vi "GetDecorationName.vi"(6 "error in":errorcluster, 9 "Decoration in":refnum<class "Decoration.lvclass">) -> (0 "error out":errorcluster, 3 "Decoration out":refnum<class "Decoration.lvclass">, 4 "name":string)   [LabVIEW 2014, in "Raspberry Pi Compatible Compiler for LabVIEW.lvlib" / "PythonConverter_GUI.lvclass"]
uses:
  PythonConverter_GUI.lvclass
  VI Interpreter/Classes/Decoration/Decoration.lvclass
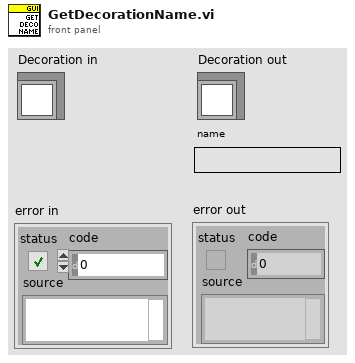
[diagram p1: front panel]
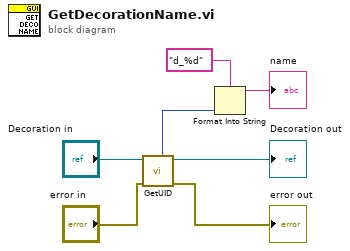
[diagram p0: block diagram]
diagram:
  n1 = call-dynamic "GetUID.vi"("error in"="error in", "GObject in"="Decoration in") -> ("error out"=→"error out":errorcluster, "GObject out"=→"Decoration out":refnum<class "Decoration.lvclass">, "UID"=w2:i32)  [unwired: 5 in]
  n2 = Format Into String(format string="d_%d", w2) -> (resulting string=→"name":string)  [unwired: 2 in, 1 out]
